vi "GUI_BacklashCompensation.vi"() -> ()   [LabVIEW 2013]
uses:
  Shared/GUI_Template/GUI_master/tcp new data cluster.ctl
  <vilib>/vision/NI_Vision_Development_Module.lvlib
  <vilib>/Analysis/NI_AALBase.lvlib
panel:
  in  "STOP Queue in":refnum<queue>
  out "Waveform Graph":dbl[](graph)=[422.8855895996094, 422.8855895996094, 422.8941345214844, 422.8941345214844, 423.1112365722656, 423.1112365722656, 422.01690673828125, 422.01690673828125, 427.6122131347656, 427.6122131347656, 471.3069763183594, 471.3069763183594, 306.5130310058594, 306.5130310058594, 391.4015197753906, 391.4015197753906, 420.5753479003906, 420.5753479003906, 421.91107177734375, 421.91107177734375, 426.7707824707031, 426.7707824707031, 423.4275207519531, 423.4275207519531, 423.1675109863281, 423.1675109863281, 423.3919677734375, 423.3919677734375, 423.0746154785156, 423.0746154785156, 423.0746154785156, 423.0746154785156, 422.84765625, 422.84765625, 422.84765625, 422.84765625, 423.07794189453125, 423.07794189453125, 423.1611328125, 423.1611328125, 423.1442565917969, 423.1442565917969, 423.1442565917969, 423.1442565917969, 423.1442565917969, 423.1442565917969, 422.7291259765625, 422.7291259765625, 422.73126220703125, 422.73126220703125, 422.7818908691406, 422.7818908691406, 422.8550109863281, 422.8550109863281, 423.06195068359375, 423.06195068359375, 423.01092529296875, 423.01092529296875, 424.062744140625, 424.062744140625, 424.00897216796875, 424.00897216796875, 423.8546142578125, 423.8546142578125, 423.6816101074219, 423.6816101074219, 422.52520751953125, 422.52520751953125, 422.9999084472656, 422.9999084472656, 422.9999084472656, 422.9261474609375, 422.9261474609375, 422.9966125488281, 422.9966125488281, 423.02850341796875, 423.02850341796875, 422.93914794921875, 422.93914794921875, 422.786376953125, 422.786376953125, 422.844482421875, 422.844482421875, 422.844482421875, 422.844482421875, 422.844482421875, 422.844482421875, 422.844482421875, 423.02191162109375, 423.02191162109375, 423.03369140625, 423.03369140625, 423.0235900878906, 423.0235900878906, 422.85675048828125, 422.85675048828125, 422.9195861816406, 422.9195861816406, 422.7881164550781, 422.7881164550781, 422.65985107421875, 422.65985107421875, 422.6369323730469, 422.6369323730469, 422.7926330566406, 422.7926330566406, 422.8153381347656, 422.8153381347656, 422.8182678222656, 422.8182678222656, 422.78759765625, 422.78759765625, 422.826416015625, 422.826416015625, 422.83441162109375, 422.83441162109375, 422.6646423339844, 422.6646423339844, 422.8706359863281, 422.8706359863281, 422.9045715332031, 422.9045715332031, 422.9270324707031, 422.9270324707031, 422.9468688964844, 422.9468688964844, 422.97906494140625, 422.97906494140625, 423.1133117675781, 423.1133117675781, 423.0961608886719, 423.0961608886719, 423.0714111328125, 423.0714111328125, 422.94146728515625, 422.94146728515625, 422.791259765625, 422.791259765625, 422.78851318359375, 422.78851318359375, 422.78851318359375, 422.8364562988281, 422.8364562988281, 422.8364562988281, 422.8364562988281, 422.8364562988281, 422.7038879394531, 422.7038879394531, 422.6075744628906, 422.6075744628906, 422.61688232421875, 422.61688232421875, 422.61688232421875, 422.61688232421875, 422.61688232421875, 422.33514404296875, 422.33514404296875, 422.7622375488281, 422.7622375488281, 422.4975280761719, 422.4975280761719, 422.533935546875, 422.533935546875, 422.52154541015625, 422.52154541015625, 422.55474853515625, 422.55474853515625, 422.6619567871094, 422.6619567871094, 422.73046875, 422.73046875, 422.70367431640625, 422.70367431640625, 422.6319885253906, 422.6319885253906, 422.8172607421875, 422.8172607421875, 422.7842102050781, 422.7842102050781, 422.79852294921875, 422.79852294921875, 422.8083801269531, 422.8083801269531, 422.8841857910156, 422.8841857910156, 422.8841857910156, 422.8841857910156, 422.8841857910156, 422.8841857910156, 422.8841857910156, 422.8892517089844, 422.8892517089844, 422.9994201660156, 422.9994201660156, 422.9523620605469, 422.9523620605469, 422.9224853515625, 422.9224853515625, 422.9607849121094, 422.9607849121094, 423.0086364746094, 423.0086364746094, 422.8628234863281, 422.8628234863281, 422.9157409667969, 422.9157409667969, 422.968505859375, 422.968505859375, 423.04376220703125, 423.04376220703125, 423.0496826171875, 423.0496826171875, 422.9351501464844, 422.9351501464844, 423.0882873535156, 423.0882873535156, 423.0077819824219, 423.0077819824219, 423.0894775390625, 423.0894775390625, 423.0082702636719, 423.0082702636719, 423.1181640625, 423.1181640625, 423.14190673828125, 423.14190673828125, 423.26397705078125, 423.26397705078125, 423.26531982421875, 423.26531982421875, 423.24371337890625, 423.24371337890625, 423.0641174316406, 423.0641174316406, 424.45123291015625, 424.45123291015625, 424.3868713378906, 424.3868713378906, 424.27752685546875, 424.27752685546875, 423.0848388671875, 423.0848388671875, 423.0848388671875, 423.0848388671875, 423.0848388671875, 423.1082763671875, 423.1082763671875, 423.31976318359375, 423.31976318359375, 423.31976318359375, 423.31976318359375, 423.0191650390625, 423.0191650390625, 423.0191650390625, 423.0191650390625, 423.30194091796875, 423.30194091796875, 423.2236633300781, 423.2236633300781, 423.13543701171875, 423.13543701171875, 423.13543701171875, 422.9753112792969, 422.9753112792969, 423.1534423828125, 423.1534423828125, 423.3553771972656, 423.3553771972656, 423.4159851074219, 423.4159851074219, 423.3205871582031, 423.3205871582031, 424.4618835449219, 424.4618835449219, 424.5314025878906, 424.5314025878906, 423.92315673828125, 423.92315673828125, 424.1344909667969, 424.1344909667969, 424.0238037109375, 424.0238037109375, 424.0238037109375, 424.0238037109375, 423.9875183105469, 423.9875183105469, 423.0684509277344, 423.0684509277344, 423.0328063964844, 423.0328063964844, 423.0791320800781, 423.0791320800781, 422.7436828613281, 422.7436828613281, 422.7146911621094, 422.7146911621094, 422.7146911621094, 422.7146911621094, 422.7146911621094, 422.7146911621094, 422.7146911621094, 422.9085998535156, 422.9085998535156, 423.1405029296875, 423.1405029296875, 423.0606689453125, 423.0606689453125, 422.82550048828125, 422.82550048828125, 422.703857421875, 422.703857421875, 422.8069152832031, 422.8069152832031, 422.392822265625, 422.392822265625, 421.67236328125, 421.67236328125, 421.4425354003906, 421.4425354003906, 421.2494812011719, 421.2494812011719, 421.2098388671875, 421.2098388671875, 421.07257080078125, 421.07257080078125, 420.8315734863281, 420.8315734863281]
  in  "clear data":bool
  in  "add data":bool
  out "Centroid":cluster{"X Centroid":sgl, "Y Centroid":sgl}={"X Centroid"=420.83157, "Y Centroid"=164.06723} {"Y Centroid" format="%.2f"; "X Centroid" format="%.2f"}
  in  "Size & Order #":T1={"X Size"=3, "Y Size"=3, "Order #"=4}
  out "image":T2(plugin-control) caption="Monitor Image (binary)"
  out "XY Graph":cluster{dbl[], dbl[]}(graph)={[1.32978, 1.33477, 1.33477, 1.32977, 1.33476], [446.65716796875, 415.2008444296347, 415.2846252441406, 420.9924057006836, 415.41217041015625]}
  in  "take data":bool=TRUE
  in  "position.Axis 2::2":dbl=3.04167 caption="y" min=0.0 max=0.0
  in  "position.Axis 1::2":dbl=1.32976 caption="x" min=0.0 max=6.0
  in  "GUIdevice 2":string="StagingTRA3"
  in  "centroidy::1":dbl=210.959686 min=0.0 max=0.0
  in  "centroidx::1":dbl=444.310547 min=0.0 max=0.0
  out "image::1":T2(plugin-control) caption="Monitor Image (binary)"
  in  "stop":bool
  in  "GUIdevice 1":string="StagingModeImager2"
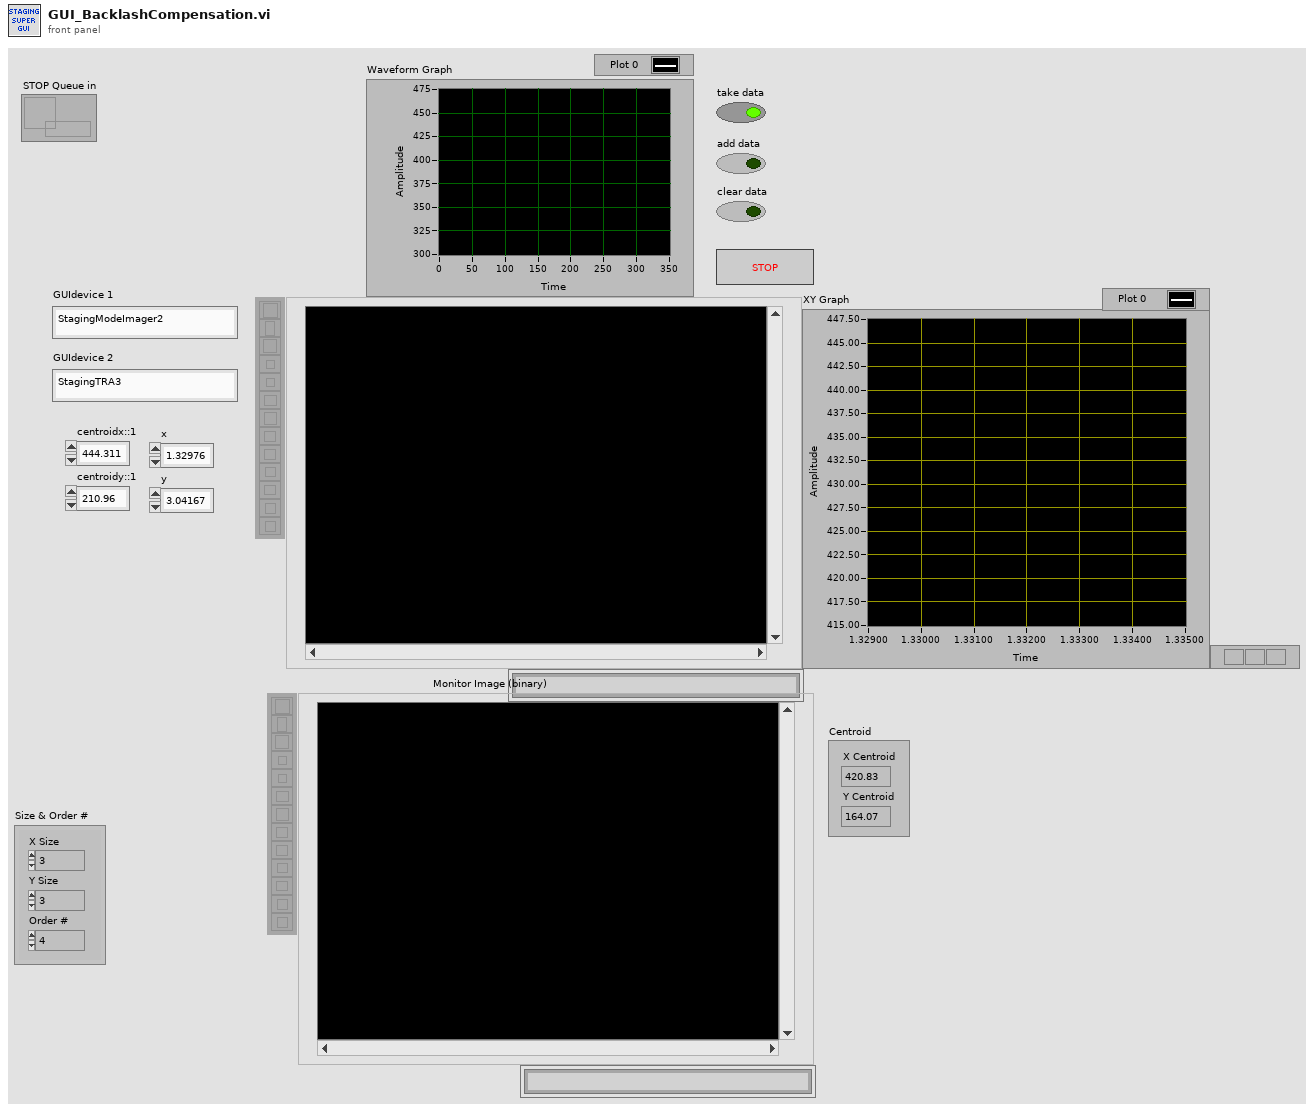
[diagram p1: front panel]
types:
  T1 = cluster{"X Size":i32, "Y Size":i32, "Order #":i32}
  T2 = typedef "IMAQ Image.ctl" = refnum<image>
  T3 = typedef "Image Type" = u32
  T4 = typedef "tcp new data cluster.ctl" = cluster{"EventEnum":enum16{"new data", "connection status update"}, "Device name":string}
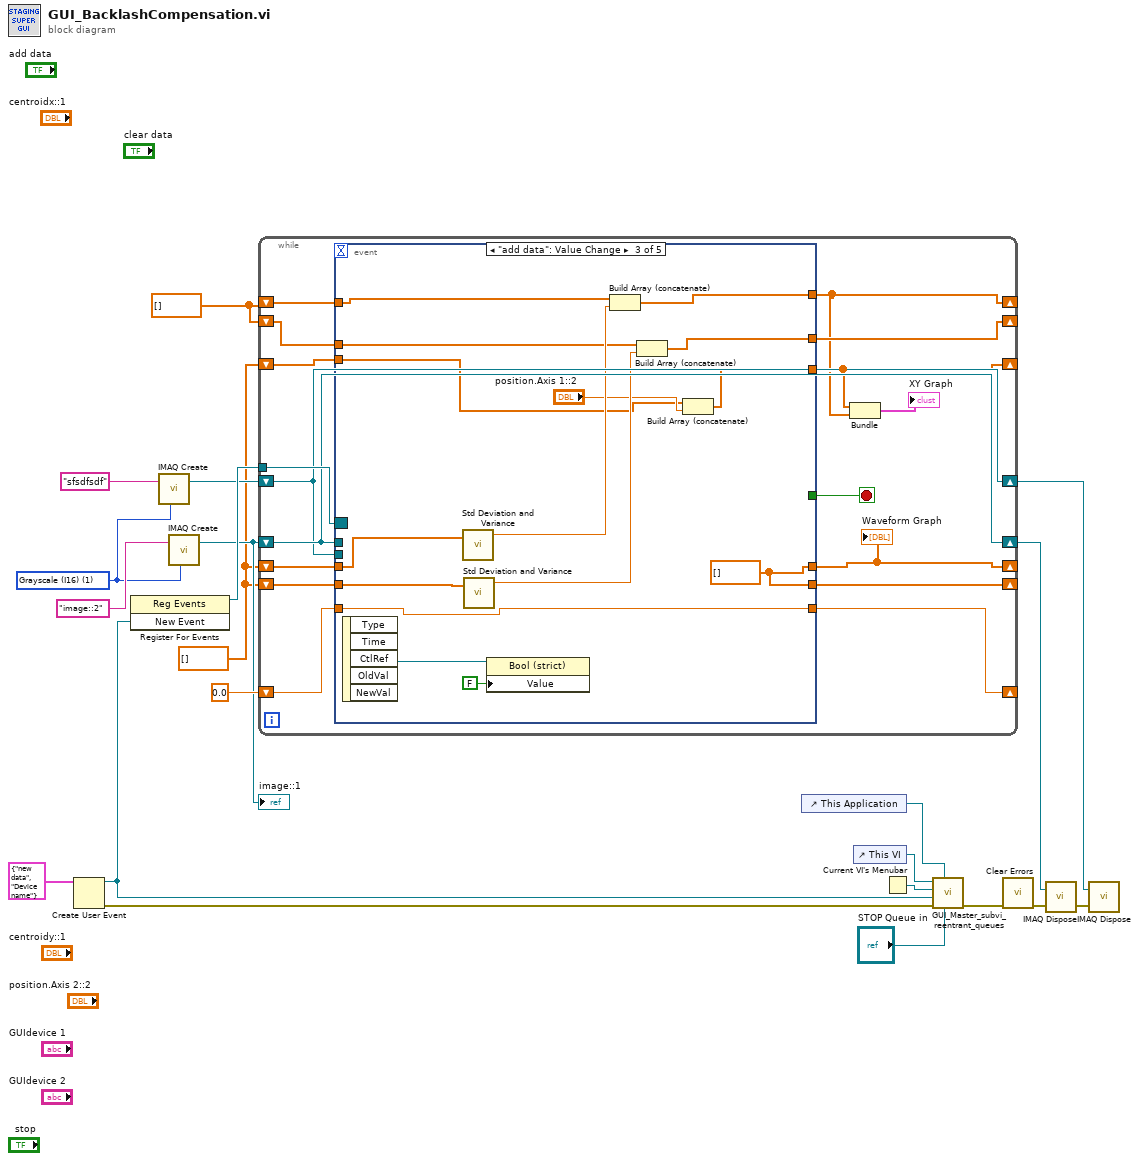
[diagram p0: block diagram]
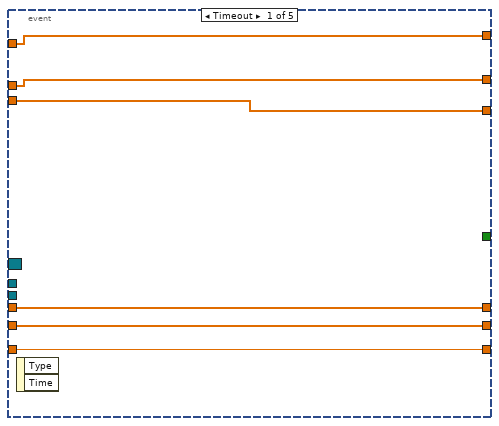
[diagram p2: hidden frame]
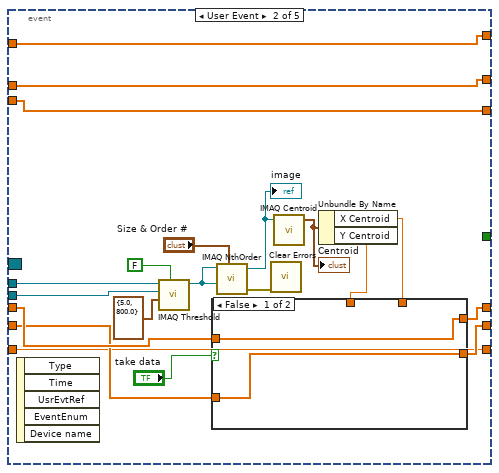
[diagram p3: hidden frame]
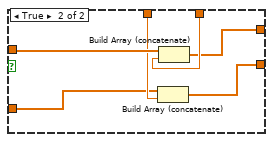
[diagram p4: hidden frame]
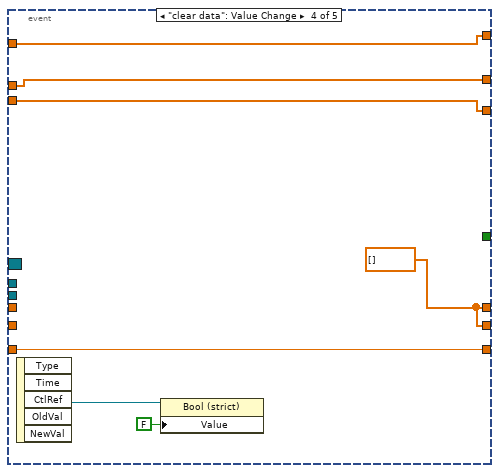
[diagram p5: hidden frame]
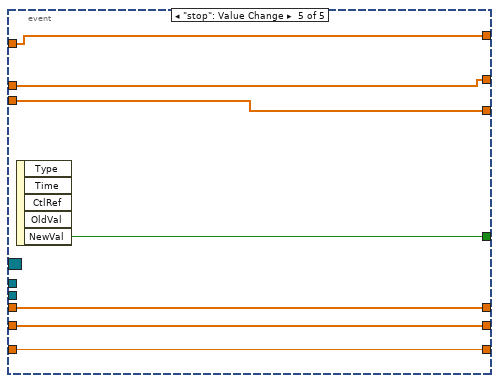
[diagram p6: hidden frame]
diagram:
  w2 = dbl[] []
  w3 = dbl[] []
  w9 = T3 1 items=["Grayscale (U8)", "Grayscale (I16)", "Grayscale (SGL)", "Complex (CSG)", "RGB (U32)", "HSL (U32)", "RGB (U64)", "Grayscale (U16)"] ("Image Type")
  n1 = Create User Event(user event datatype=T4 {"EventEnum"=enum."new data", "Device name"="Device name"} ("New Event")) -> (user event=w18:refnum<user-event>, error out=w20:errorcluster)  [unwired: 1 in]
  n2 = register-events(w18) -> (reference out=w17:refnum<event-registration>)  [unwired: 2 in, 1 out]
  n3 = call "IMAQ Create"("Image Name"="sfsdfsdf", "Image Type"=w9) -> ("New Image"=w7:T2)  [unwired: 3 in, 1 out]
  n4 = call "IMAQ Create"("Image Name"="image::2", "Image Type"=w9) -> ("New Image"=w4:T2)  [unwired: 3 in, 1 out]
  "image::1" <- w4
  n5 = while {
    tunnel: w17 -> [w38]
    shift-right: [w35] -> _
    shift-left: 0.0 -> [w36]
    shift-right: [w32] -> _
    shift-left: w3 -> [w33]
    shift-right: [w23] -> _
    shift-left: w3 -> [w34]
    shift-right: [w30] -> w14
    shift-left: w4 -> [w30]
    shift-right: [w29] -> w6
    shift-left: w7 -> [w29]
    shift-right: [w28] -> _
    shift-left: w3 -> [w27]
    shift-right: [w22] -> _
    shift-left: w2 -> [w26]
    shift-right: [w24] -> _
    shift-left: w2 -> [w25]
    stop <- w37 stop-if-true
    n6 = event shown="[2] \"add data\": Value Change" {
      selector: w38 -> [_ _ _ _ _]
      dyn-events: _ -> [_ _ _ _ _]
      timeout: _ -> [_ _ _ _ _]
      tunnel: [_ _ _ _ w101] -> w37
      tunnel: w36 -> [w44 w46 w74 w89 w100]
      tunnel: [w44 w46 w74 w89 w100] -> w35
      tunnel: [w42 w52 w73 w90 w98] -> w32
      tunnel: [w43 w45 w75 w88 w99] -> w23
      tunnel: w34 -> [w43 w45 w76 w88 w99]
      tunnel: w33 -> [w42 w54 w87 _ w98]
      tunnel: w30 -> [_ w61 _ _ _]
      tunnel: w29 -> [_ w62 _ _ _]
      tunnel: [w41 w50 w73 w90 w97] -> w28
      tunnel: w27 -> [w41 w49 w86 _ w97]
      tunnel: w26 -> [w40 w48 w84 w92 w96]
      tunnel: [w40 w48 w83 w92 w96] -> w22
      tunnel: w25 -> [w39 w47 w82 w91 w95]
      tunnel: [w39 w47 w80 w91 w95] -> w24
      event Timeout {
        n7 = event-data() -> ()  [unwired: 1 in, 2 out]
      }
      event User Event {
        n8 = event-data() -> ()  [unwired: 1 in, 5 out]
        n9 = call "IMAQ Threshold"("Keep/Replace Value (Replace)"=FALSE, "Range"=cluster{"Lower value":sgl, "Upper value":sgl} {"Lower value"=5.0, "Upper value"=800.0}, "Image Dst"=w62, "Image Src"=w61) -> ("Image Dst Out"=w60:T2)  [unwired: 6 in, 1 out]
        n10 = call "IMAQ NthOrder"("Image Src"=w60, "Size & Order #"="Size & Order #", "Image Dst"=w60) -> ("Image Dst Out"=w57:T2, "error out"=w58:errorcluster)  [unwired: 4 in]
        "image" <- w57
        n11 = call <vilib>:"Clear Errors.vi"("error in (no error)"=w58) -> ()  [unwired: 6 in, 1 out]
        n12 = call "IMAQ Centroid"("Image"=w57) -> ("Centroid"=w56:cluster{"X Centroid":sgl, "Y Centroid":sgl})  [unwired: 3 in, 1 out]
        "Centroid" <- w56
        n13 = Unbundle By Name(w56) -> ("X Centroid"=w53:sgl, "Y Centroid"=w51:sgl)
        n14 = case shown="False" "take data" {
          tunnel: w54 -> [w66 w72]
          tunnel: w53 -> [_ w71]
          tunnel: [w66 w70] -> w52
          tunnel: w51 -> [_ w69]
          tunnel: [w65 w68] -> w50
          tunnel: w49 -> [w65 w67]
          frame False {
          }
          frame True {
            n15 = Build Array (concatenate)(w67, w69) -> (w68:dbl[])
            n16 = Build Array (concatenate)(w72, w71) -> (w70:dbl[])
          }
        }
      }
      event "add data": Value Change {
        w73 = dbl[] []
        n17 = event-data() -> ("CtlRef"=w79:refnum<vi>)  [unwired: 1 in, 4 out]
        n18 = call <vilib>:"Std Deviation and Variance.vi"("X"=w87) -> ("mean"=w85:dbl)  [unwired: 1 in, 2 out]
        n19 = call <vilib>:"Std Deviation and Variance.vi"("X"=w86) -> ("mean"=w81:dbl)  [unwired: 1 in, 2 out]
        n20 = property class="Bool (strict)"(reference=w79, "Value"=FALSE) -> ()  [unwired: 1 in, 2 out]
        n21 = Build Array (concatenate)(w84, w85) -> (w83:dbl[])
        n22 = Build Array (concatenate)(w82, w81) -> (w80:dbl[])
        n23 = Build Array (concatenate)(w76, "position.Axis 1::2") -> (w75:dbl[])
      }
      event "clear data": Value Change {
        w90 = dbl[] []
        n24 = event-data() -> ("CtlRef"=w94:refnum<vi>)  [unwired: 1 in, 4 out]
        n25 = property class="Bool (strict)"(reference=w94, "Value"=FALSE) -> ()  [unwired: 1 in, 2 out]
      }
      event "stop": Value Change {
        n26 = event-data() -> ("NewVal"=w101:bool)  [unwired: 1 in, 4 out]
      }
    }
    "Waveform Graph" <- w32
    n27 = Bundle(w23, w22) -> (→"XY Graph":cluster{dbl[], dbl[]})  [unwired: 1 in]
  }
  n28 = control-ref of="This Application"() -> (w10:refnum<vi>)
  n29 = control-ref of="This VI"() -> (w12:refnum<vi>)
  n30 = Current VI's Menubar() -> (w11:refnum<k9>)
  n31 = call "GUI_Master_subvi_reentrant_queues.vi"("STOP Queue in"="STOP Queue in", "This Application"=w10, "error in (no error)"=w20, "tcp data event"=w18, "Caller menu reference"=w11, "Caller VI ref"=w12) -> ("error out"=w19:errorcluster)  [unwired: 5 in]
  n32 = call <vilib>:"Clear Errors.vi"("error in (no error)"=w19) -> ("error out"=w13:errorcluster)  [unwired: 6 in]
  n33 = call "IMAQ Dispose"("Image"=w14, "error in (no error)"=w13) -> ("error out"=w5:errorcluster)  [unwired: 4 in]
  n34 = call "IMAQ Dispose"("Image"=w6, "error in (no error)"=w5) -> ()  [unwired: 4 in, 1 out]
